vi "File Stream.vi"() -> ()   [LabVIEW 2014]
doc: "If you want to read a video from your hdd, you can use the functionality of the file stream.\nAfter a stream is initialized from the file, the images are read continuously."
uses:
  MSC Video_class/MSC Video.lvclass
  MSC Image_class/MSC Image.lvclass
panel:
  out "Frame Number":i32
  in  "Path":path=path "Browse for Path ->"
  out "error out":errorcluster
  in  "stop":bool
  out "Live Image":picture
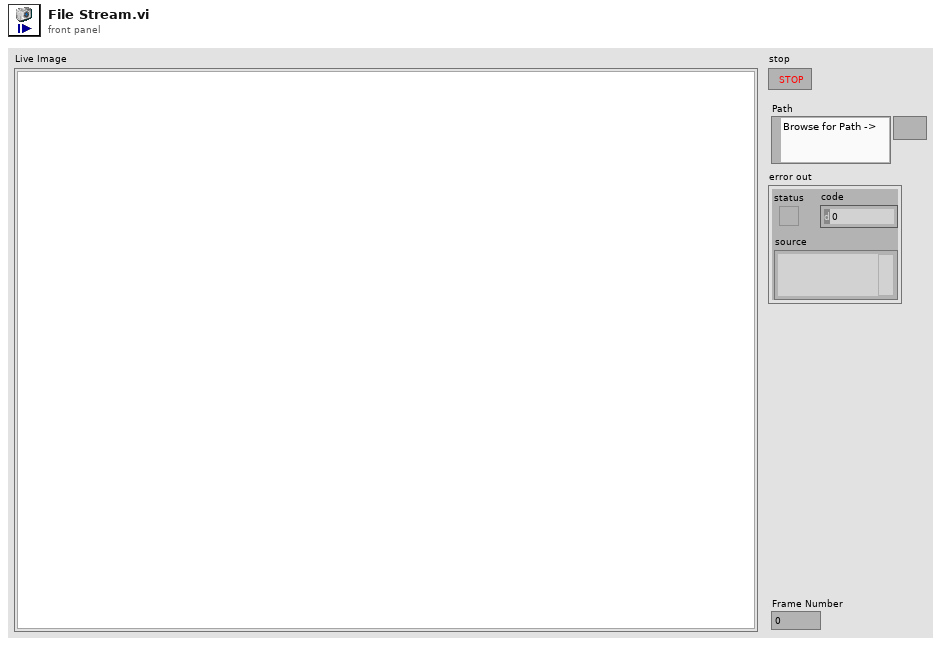
[diagram p1: front panel]
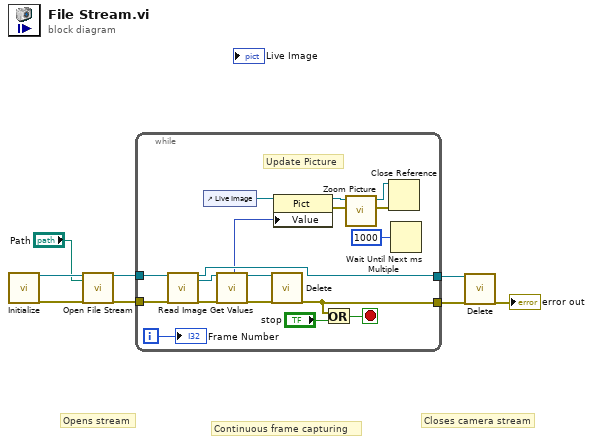
[diagram p0: block diagram]
diagram:
  # "Closes camera stream"
  # "Continuous frame capturing"
  # "Opens stream"
  n1 = call "Initialize.vi"() -> ("video out"=w5:refnum<class "MSC Video.lvclass">, "error out"=w4:errorcluster)  [unwired: 18 in]
  n2 = call-dynamic "Open File Stream.vi"("video in"=w5, "File Path"="Path", "error in (no error)"=w4) -> ("video out"=w2:refnum<class "MSC Video.lvclass">, "error out"=w1:errorcluster)  [unwired: 15 in]
  n3 = while {
    tunnel: w2 -> [w26]
    tunnel: w1 -> [w25]
    tunnel: [w23] -> w8
    tunnel: [w17] -> w7
    i -> [w9]
    stop <- w24 stop-if-true
    # "Update Picture"
    n4 = call-dynamic "Read Image.vi"("video in"=w26, "error in (no error)"=w25) -> ("video out"=w23:refnum<class "MSC Video.lvclass">, "image out"=w22:refnum<class "MSC Image.lvclass">, "error out"=w21:errorcluster)  [unwired: 15 in]
    n5 = control-ref of="Live Image"() -> (w16:refnum<vi>)
    n6 = call-dynamic "Get Values.vi"("image in"=w22, "error in (no error)"=w21) -> ("picture"=w11:picture, "image out"=w19:refnum<class "MSC Image.lvclass">, "error out"=w18:errorcluster)  [unwired: 10 in, 5 out]
    n7 = call-dynamic "Delete.vi"("image in"=w19, "error in (no error)"=w18) -> ("error out"=w17:errorcluster)  [unwired: 17 in]
    n8 = property class="Pict"(reference=w16, "Value"=w11) -> (reference out=w12:refnum<vi>, error out=w13:errorcluster)  [unwired: 1 in]
    n9 = Or(x=w17, y="stop") -> (x .or. y?=w24:bool)
    n10 = call "Zoom Picture.vi"("error in (no error)"=w13, "Picture in"=w12) -> ("error out"=w15:errorcluster, "Picture out"=w14:refnum<vi>)  [unwired: 8 in]
    n11 = Close Reference(reference=w14, error in (no error)=w15) -> ()  [unwired: 1 out]
    n12 = Wait Until Next ms Multiple(millisecond multiple=u32 1000) -> ()  [unwired: 1 out]
    "Frame Number" <- w9
  }
  n13 = call-dynamic "Delete.vi"("video in"=w8, "error in (no error)"=w7) -> ("error out"=→"error out":errorcluster)  [unwired: 17 in]
